vi "DevelopRecipe.vi"(9 "Flappy Velocity":dbl format="%#_13g", 10 "Flappy Height":dbl format="%#_13g", 11 "Pipe location (left, top)":dbl[](array[numeric])) -> (3 "Recipe":T1[](array[typedef]))   [LabVIEW 2014]
uses:
  Recipe step.ctl
  STD - Tap Mode.ctl
  Globals.vi
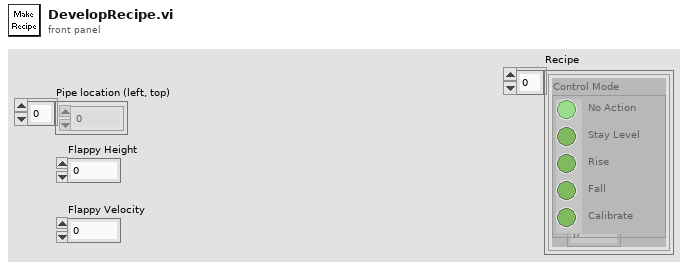
[diagram p1: front panel]
types:
  T1 = typedef "Recipe step.ctl" = cluster{"Control Mode":T2, "Length (s)":dbl}
  T2 = typedef "STD - Tap Mode.ctl" = enum32{"No Action", "Stay Level", "Rise", "Fall", "Calibrate"}
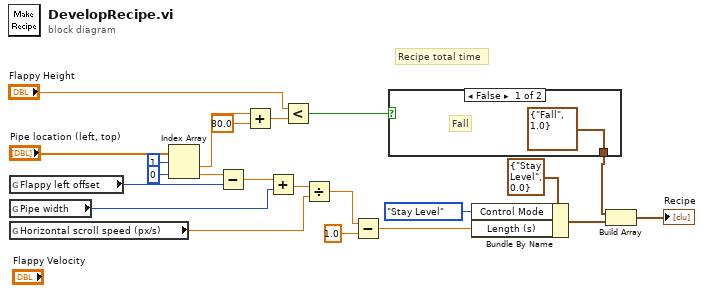
[diagram p0: block diagram]
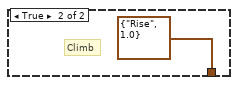
[diagram p2: hidden frame]
diagram:
  # "Recipe total time"
  n1 = global read "Globals.vi" "Flappy left offset"() -> (w21:u32)
  n2 = global read "Globals.vi" "Pipe width"() -> (w19:u32)
  n3 = global read "Globals.vi" "Horizontal scroll speed (px/s)"() -> (w17:dbl)
  n4 = Index Array(array="Pipe location (left, top)", index #1=1 ("index"), index #2=0 ("index")) -> (element #1=w8:dbl, element #2=w9:dbl)
  n5 = Subtract(x=w9, y=w21) -> (x-y=w20:dbl)
  n6 = Add(x=w8, y=80.0) -> (x+y=w5:dbl)
  n7 = Add(x=w20, y=w19) -> (x+y=w18:dbl)
  n8 = Less?(x="Flappy Height", y=w5) -> (x < y?=w3:bool)
  n9 = Divide(x=w18, y=w17) -> (x/y=w14:dbl)
  n10 = Subtract(x=w14, y=1.0) -> (x-y=w13:dbl)
  n11 = case shown="False" w3 {
    tunnel: [T1 {"Control Mode"=enum."Fall", "Length (s)"=1.0} ("Recipe step") T1 {"Control Mode"=enum."Rise", "Length (s)"=1.0} ("Recipe step")] -> w2
    frame False {
      # "Fall"
    }
    frame True {
      # "Climb"
    }
  }
  n12 = Bundle By Name(cluster=T1 {"Control Mode"=enum."Stay Level", "Length (s)"=0.0} ("Recipe step"), "Control Mode"=STD_-_Tap_Mode."Stay Level", "Length (s)"=w13) -> (w12:T1)
  n13 = Build Array(w2, w12) -> (→"Recipe":T1[])
